vi "LIDARBrake - Rev3.vi"() -> ()   [LabVIEW 2018]
uses:
  PWFusion_TimeOfFlight_SEN-36005/LabVIEW-FRC/ToF_TypeDef/PwF ToF RangingMode.ctl
  <vilib>/Platform/TimedLoop/XDataNode/timing_clust.ctl
  <vilib>/Platform/TimedLoop/XDataNode/nitl_modes.ctl
  <vilib>/Platform/TimedLoop/XDataNode/wakeup.ctl
  <userlib>/836-Library/System/TDMS_V2/Support/TDMS_DevRef.ctl
  <userlib>/836-Library/System/TDMS_V2/Support/Logging_Settings.ctl
  <userlib>/836-Library/System/TDMS_V2/Support/Group_FIFO_Config.ctl
  <userlib>/836-Library/System/TDMS_V2/Support/Channel_FIFO_Config.ctl
  <vilib>/addons/control/pid/pid.llb/PID (DBL).vi
  <vilib>/platform/TimedLoop/XDataNode/XDataNode.xnode
  <vilib>/Platform/TimedLoop/XDataNode/XDNodeRunTimeDep.lvlib
  <vilib>/addons/control/pid/NI_PID_pid.lvlib
panel:
  out "RangingStatus":u8
  in  "LIDAR CF":dbl=1.0
  in  "x":dbl=-56.0
  in  "Reset 2":bool=TRUE
  out "Diag 2":cluster{dbl, dbl, i16}(graph)={-218.49922960069443, 18.330708661417322, 0}
  in  "Reset":bool=TRUE
  out "Diag":cluster{i32, i16, dbl, i16}(graph)={1, 0, 4.5, 0}
  in  "Read Enable":T1={"Cal Status"=TRUE, "Orientation"=TRUE, "Gyro"=FALSE, "Accelerometer"=FALSE, "Quanterion"=FALSE, "Accel Mode"=enum."Linear", "Magnetometer"=FALSE, "Register Mode"=enum."Quaternion"}
  in  "Tab Control":enum32{"Sonar", "LIDAR"}(tab)=enum."LIDAR"
  in  "Tol (sec)":dbl=0.25 format="%#_13g"
  in  "Tol (in)":dbl=1.1
  out "Arrived":bool
  out "Sonar Error":dbl=-3.3307086614173222
  in  "Rate Thresh":dbl=100.0 format="%#_13g"
  out "OOR":bool
  out "Mode":bool=TRUE
  in  "hi limit":dbl=200.0
  out "Strobe":bool
  in  "standoff":dbl=15.0 format="%.2f"
  out "Sonar Left":cluster{"Filtered":dbl, dbl}(graph)={"Filtered"=18.330708661417322, 18.330708661417322}
  out "LIDAR Late?":bool
  out "Period":i64=60
  in  "Reset Enc":bool
  out "Enc":dbl=162.49922960069443
  in  "Hyster":dbl=0.1 format="%#_13g"
  out "State":i32=1
  in  "reset IMU":bool
  in  "Test?":bool=TRUE
  in  "clamp":cluster{"output high":dbl, "output low":dbl}={"output high"=1.0, "output low"=-1.0} {"output low" format="%.2f"; "output high" format="%.2f"}
  in  "Trans":dbl=30.0
  out "close":bool=TRUE
  in  "PID Sonar":T2={"proportional gain (Kc)"=0.035, "integral time (Ti, min)"=0.0, "derivative time (Td, min)"=0.001} {"derivative time (Td, min)" format="%.5f"; "integral time (Ti, min)" format="%.3f"; "proportional gain (Kc)" format="%.3f"}
  in  "Use Enc?":bool
  out "Sonar PID":cluster{"setpoint":dbl, "Filtered":dbl, i16}(graph)={"setpoint"=15.0, "Filtered"=60.0, 0}
  out "PID error":dbl=45.0
  in  "scale enc":dbl=-0.04
  in  "db":dbl
  out "Inches 2":dbl(slide)=18.330708661417322 scale=0.0..90.0
  out "Inches":dbl(slide)=18.330708661417322 scale=0.0..90.0
  out "LIDAR (in)":dbl=18.330708661417322
  out "State 2":i32=1
  out "LIDAR Stable":bool
  in  "LIDAR Stable 2":dbl format="%#_13g"
  in  "Desired  Sample Rate ms 2":u16=50
  in  "Desired Range Mode 2":T3=enum."Medium (2m)"
  in  "RS LIDAR":bool
  in  "threshold":dbl=10.0 format="%#_13g"
  # "Real Time Data Repair"
  # "Pre-Filter"
  # "Post-Filter"
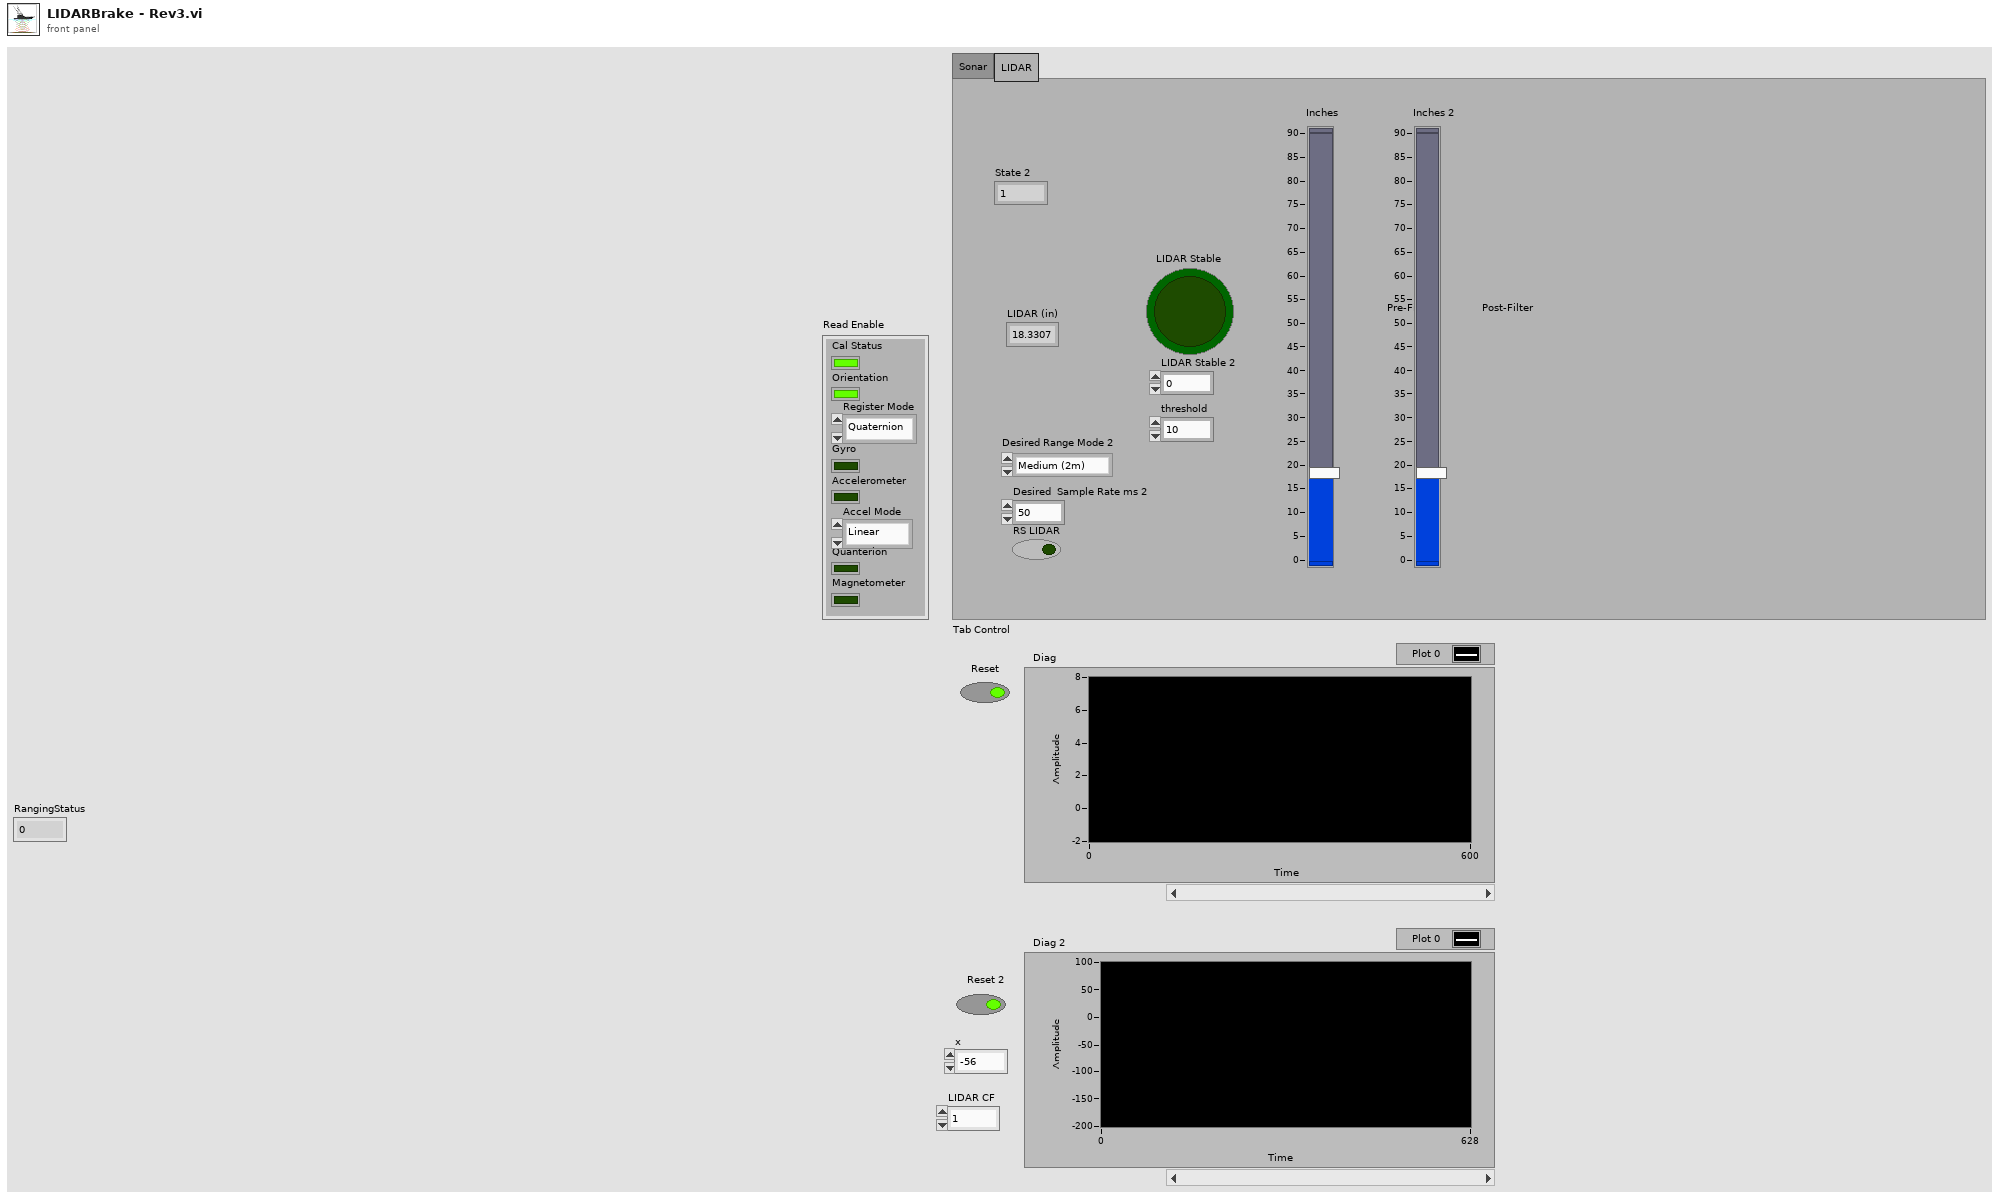
[diagram p1: front panel]
types:
  T1 = cluster{"Cal Status":bool, "Orientation":bool, "Gyro":bool, "Accelerometer":bool, "Quanterion":bool, "Accel Mode":enum8{"Raw Data", "Linear", "Gravity"}, "Magnetometer":bool, "Register Mode":enum8{"Euler", "Quaternion"}}
  T2 = cluster{"proportional gain (Kc)":dbl, "integral time (Ti, min)":dbl, "derivative time (Td, min)":dbl}
  T3 = typedef "PwF ToF RangingMode.ctl" = enum8{"Short (1.3m)", "Medium (2m)", "Long (4m)"}
  T4 = typedef "ImuDevRef.ctl" = cluster{"I2CDevRef":T5, "Valid Cal File?":bool}
  T5 = typedef "WPI_I2CDevRef.ctl" = cluster{"DevStatus":errorcluster, "Device Address":u8, "Handle":i32, "I2C Bus":T6}
  T6 = typedef "i2c_bus.ctl" = enum16{"I2C On-Board", "I2C MXP", "Invalid"}
  T7 = typedef "XDNodeRunTimeDep.lvlib/timing_clust.ctl" = cluster{"Expected End [f-1]":u64, "Actual End [f-1]":u64, "Finished Late? [f-1]":bool, "Expected End [i-1]":u64, "Actual End [i-1]":u64, "Finished Late? [i-1]":bool, "Expected Start [i]":u64, "Actual Start [i]":u64, "Expected Start [f]":u64, "Actual Start [f]":u64, "Source Name":string, "Structure Name":string, "Period":i64, "Deadline":i64, "Offset":i64, "Start":i64, "Priority":i32, "Timeout":i32, "Mode":T8, "Wakeup Reason":T9, "Error":errorcluster, "Source Type":string, "Secondary Source Type":string, "Global End Time":u64, "Global Start Time":u64, "Frame Duration":u64, "Iteration Duration":u64, "Assigned CPU":i32, "I/O Scan Engine Mode":u32}
  T8 = typedef "XDNodeRunTimeDep.lvlib/nitl_modes.ctl" = enum32{"No Change", "Process missed periods, maintain original phase", "Discard missed periods, maintain original phase", "Process missed periods, ignore original phase", "Discard missed periods, ignore original phase"}
  T9 = typedef "XDNodeRunTimeDep.lvlib/wakeup.ctl" = enum32{"Normal", "Aborted", "Asynchronous wakeup", "Timing source error", "Timed loop error", "Timeout"}
  T10 = typedef "PwF ToF Ref.ctl" = cluster{"Device ID":u8, "Ranging Mode":T3, "RefNumName":string}
  T11 = typedef "TDMS_DevRef.ctl" = cluster{"Name":string, "File Ref":refnum<k34>, "Start Time":timestamp, "Logging Settings":T12, "Group FIFO Config":T13[], "Data To Write":refnum<data-value>, "semaphore":T15, "Ref Time Reset":refnum<k4>}
  T12 = typedef "Logging_Settings.ctl" = cluster{"Data Grab Period":dbl, "File Write Period":dbl, "Max Stored Size":dbl, "Burst Size":dbl}
  T13 = typedef "Group_FIFO_Config.ctl" = cluster{"Group":string, "Channels":T14[], "Channel Names":string[]}
  T14 = typedef "Channel_FIFO_Config.ctl" = cluster{"Channel":string, "FIFO":refnum<k33>}
  T15 = typedef "Semaphore RefNum" = refnum<k1>
  T16 = cluster{"Yaw":dbl, "Roll":dbl, "Pitch":dbl, "Yaw Wind":dbl, "Roll Wind":dbl, "Pitch Wind":dbl}
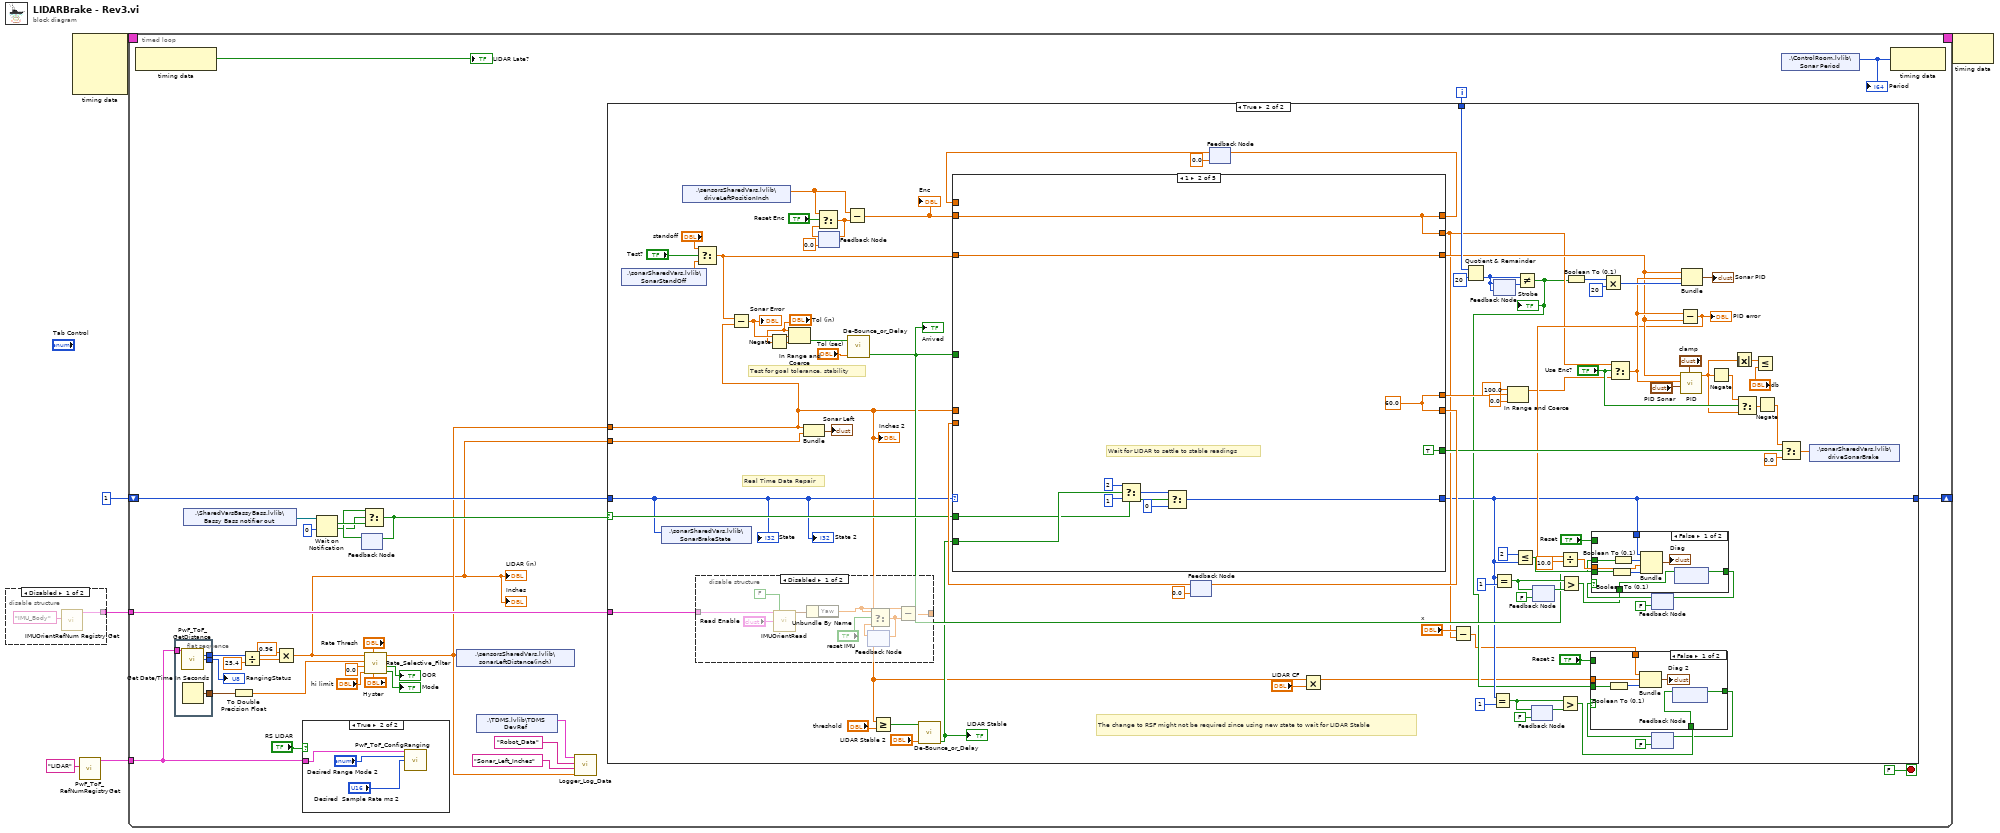
[diagram p0: block diagram]
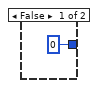
[diagram p4: hidden frame]
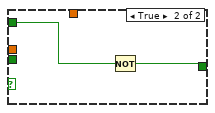
[diagram p5: hidden frame]
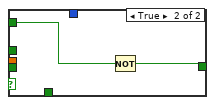
[diagram p6: hidden frame]
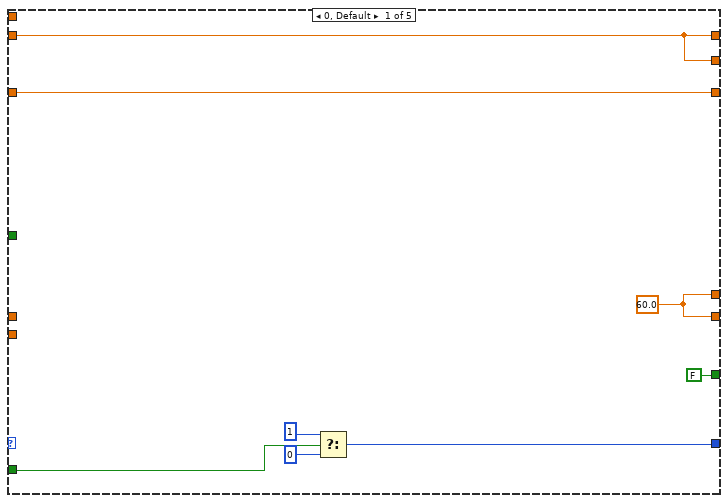
[diagram p8: hidden frame]
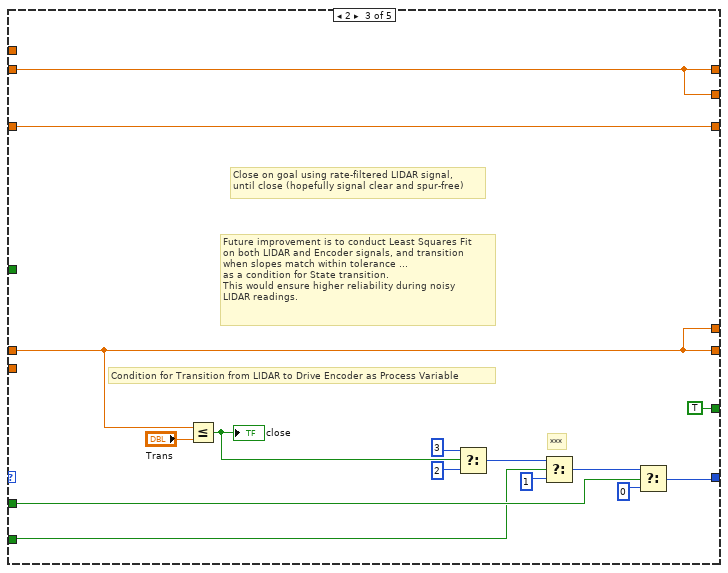
[diagram p9: hidden frame]
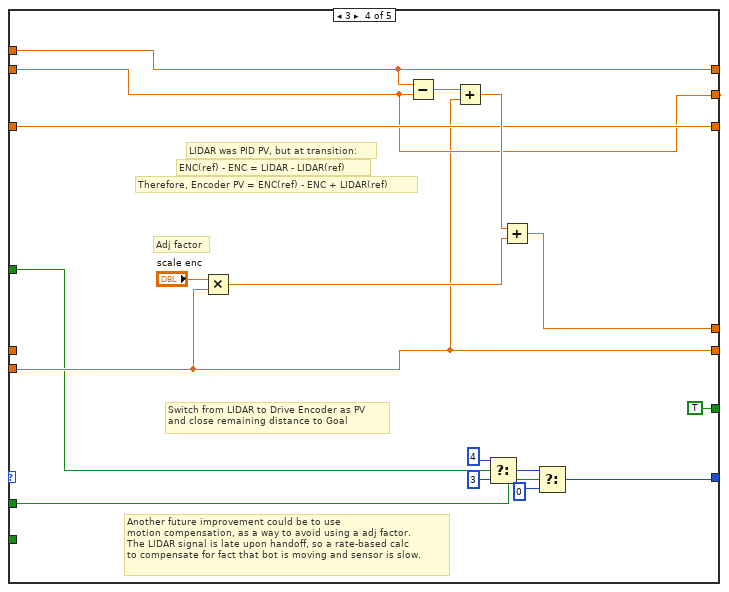
[diagram p10: hidden frame]
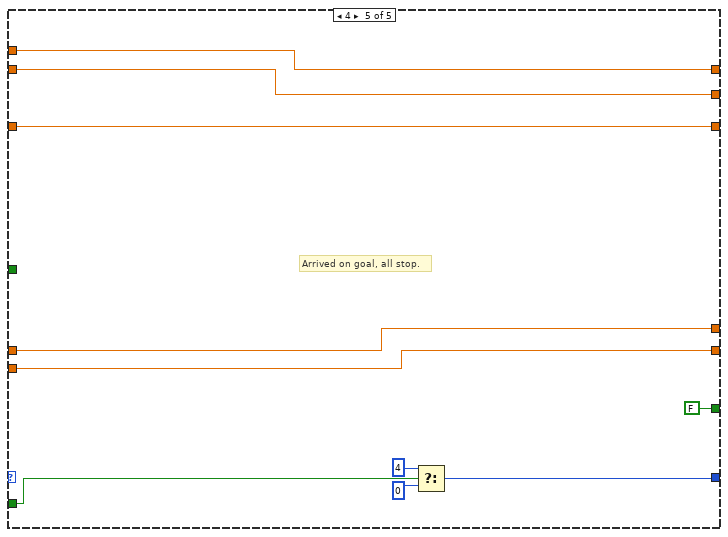
[diagram p11: hidden frame]
diagram:
  n1 = disable-structure shown="Disabled" {
    disable-tunnel: [w7 _] -> w3
    frame Disabled {
      n2 = call <userlib>:"IMUOrientRefNum Registry Get.vi"("refnum name"="IMU_Body") -> ("IMUDevRef out"=w7:T4)  [unwired: 9 in, 1 out]
    }
    frame Enabled {
    }
  }
  n3 = node-c288() -> (w6:T7)  [unwired: 4 in]
  n4 = call "PwF_ToF_RefNumRegistryGet.vi"("refnum name"="LIDAR") -> ("PwF ToF Ref"=w1:T10)  [unwired: 9 in, 1 out]
  n5 = timed-loop {
    timing: w6 -> [_]
    timing-out: [_] -> w5
    shift-right: [w35] -> _
    shift-left: 1 -> [w36]
    tunnel: w3 -> [w37]
    tunnel: w1 -> [w22]
    i -> [w39]
    stop <- FALSE stop-if-true
    n6 = node-c288() -> (→"LIDAR Late?":bool)  [unwired: 1 in]
    n7 = flat-sequence {
      tunnel: [w45] -> w27
      tunnel: [w44] -> w26
      tunnel: w22 -> [w43]
      tunnel: [w42] -> w18
      frame #0 {
        n8 = call "PwF_ToF_GetDistance.vi"("PwF ToF Ref"=w43) -> ("Dist_mm"=w44:u16, "RangingStatus"=w45:u8)  [unwired: 9 in, 4 out]
        n9 = Get Date/Time In Seconds() -> (seconds since 1Jan1904=w42:timestamp)
      }
    }
    n10 = shared-variable ".\\SharedVarsBassyBass.lvlib\\Bassy Bass notifier out"() -> (w34:refnum<notifier>)  [unwired: 1 in, 1 out]
    n11 = To Double Precision Float(number=w18) -> (double precision float=w11:dbl)
    n12 = Divide(x=w26, y=25.4) -> (x/y=w24:dbl)
    n13 = Multiply(x=0.96, y=w24) -> (x*y=w9:dbl)
    "LIDAR (in)" <- w9
    "Inches" <- w9
    n14 = case shown="True" "RS LIDAR" {
      tunnel: w22 -> [_ w46]
      frame False {
      }
      frame True {
        n15 = call "PwF_ToF_ConfigRanging.vi"("PwF ToF Ref"=w46, "Ranging Mode"="Desired Range Mode 2", "Tsamp_ms"="Desired  Sample Rate ms 2") -> ()  [unwired: 11 in, 2 out]
      }
    }
    n16 = Wait on Notification(notifier=w34, timeout in ms (-1)=0) -> (notification=w32:bool, timed out?=w30:bool)  [unwired: 2 in, 2 out]
    n17 = feedback #1() -> (w31:bool)  [unwired: 1 in]
    n18 = Select(t=w31, s=w30, f=w32) -> (s? t:f=w29:bool)
    n19 = feedback-in #1(w29) -> ()
    n20 = call <userlib>:"Rate_Selective_Filter.vi"("Hyster"="Hyster", "Rate Thresh"="Rate Thresh", "hi limit"="hi limit", "lo limit"=0.0, "Time"=w11, "Distance"=w9) -> ("Mode"=→"Mode":bool, "OOR"=→"OOR":bool, "Filtered"=w10:dbl)  [unwired: 1 in]
    n21 = shared-variable ".\\sensorsSharedVars.lvlib\\sonarLeftDistance(inch)"(w10) -> ()  [unwired: 1 in, 1 out]
    n22 = shared-variable ".\\TDMS.lvlib\\TDMS DevRef"() -> (w19:T11)  [unwired: 1 in, 1 out]
    n23 = call <userlib>:"Logger_Log_Data.vi"("Data"=w10, "Channel"="Sonar_Left_Inches", "Group"="Robot_Data", "TDMS DevRef"=w19) -> ()  [unwired: 7 in, 1 out]
    n24 = case shown="True" w29 {
      selector: w29 -> [_ w85]
      tunnel: w39 -> [_ w134]
      tunnel: w37 -> [_ w125]
      tunnel: w36 -> [_ w57]
      tunnel: [0 ("t") w62] -> w35
      tunnel: w10 -> [_ w52]
      tunnel: w9 -> [_ w51]
      frame False {
      }
      frame True {
        # "The change to RSF might not be required since using new state to wait for LIDAR Stable"
        # "Real Time Data Repair"
        # "Test for goal tolerance, stability"
        n25 = shared-variable ".\\sonarSharedVars.lvlib\\SonarStandOff"() -> (w123:dbl)  [unwired: 1 in, 1 out]
        n26 = shared-variable ".\\sonarSharedVars.lvlib\\SonarBrakeState"(w57) -> ()  [unwired: 1 in, 1 out]
        n27 = shared-variable ".\\sensorsSharedVars.lvlib\\driveLeftPositionInch"() -> (w78:dbl)  [unwired: 1 in, 1 out]
        n28 = disable-structure shown="Disabled" {
          disable-tunnel: w125 -> [w159 _]
          disable-tunnel: [w158 _] -> _
          frame Disabled {
            n29 = call <userlib>:"IMUOrientRead.vi"("IMU Dev Ref"=w159, "Orient Reset (Wind)"=FALSE, "Read Enable"="Read Enable") -> ("Orient Y/R/P"=w164:T16)  [unwired: 5 in, 7 out]
            n30 = Unbundle By Name(w164) -> ("Yaw"=w160:dbl)
            n31 = feedback #2() -> (w163:dbl)  [unwired: 1 in]
            n32 = Select(t=w160, s="reset IMU", f=w163) -> (s? t:f=w162:dbl)
            n33 = feedback-in #2(w162) -> ()
            n34 = Subtract(x=w160, y=w162) -> (x-y=w158:dbl)
          }
          frame Enabled {
          }
        }
        n35 = Select(t="standoff", s="Test?", f=w123) -> (s? t:f=w79:dbl)
        n36 = Subtract(x=w79, y=w52) -> (x-y=w133:dbl)
        "Sonar Error" <- w133
        n37 = Negate(x="Tol (in)") -> (-x=w132:dbl)
        n38 = In Range and Coerce(upper limit="Tol (in)", x=w133, lower limit=w132) -> (In Range?=w80:bool)  [unwired: 1 out]
        n39 = Bundle("Filtered"=w52, w51) -> (→"Sonar Left":cluster{"Filtered":dbl, dbl})  [unwired: 1 in]
        n40 = feedback #3(0.0) -> (w128:dbl)
        n41 = Select(t=w78, s="Reset Enc", f=w128) -> (s? t:f=w126:dbl)
        n42 = feedback-in #3(w126) -> ()
        n43 = Subtract(x=w78, y=w126) -> (x-y=w127:dbl)
        "Enc" <- w127
        n44 = call <userlib>:"De-Bounce_or_Delay.vi"("Eval Period (sec)"="Tol (sec)", "Signal Input"=w80) -> ("Stable"=w81:bool)  [unwired: 9 in]
        "Arrived" <- w81
        n45 = Greater Or Equal?(x=w52, y="threshold") -> (x >= y?=w55:bool)
        n46 = call <userlib>:"De-Bounce_or_Delay.vi"("Eval Period (sec)"="LIDAR Stable 2", "Signal Input"=w55) -> ("Stable"=w54:bool)  [unwired: 9 in]
        "LIDAR Stable" <- w54
        n47 = feedback #4(0.0 ("Filtered")) -> (w107:dbl)
        n48 = feedback #5(0.0) -> (w110:dbl)
        n49 = case shown="1" w57 {
          tunnel: [w173 w184 w200 w216 w219] -> w62
          tunnel: w85 -> [w171 w179 w199 w215 w218]
          tunnel: w79 -> [w170 w177 w194 w206 w224]
          tunnel: w127 -> [w168 w176 w192 w205 w225]
          tunnel: w52 -> [_ _ w191 _ w223]
          tunnel: w81 -> [_ _ _ w202 _]
          tunnel: [w168 w176 w192 w207 w226] -> w112
          tunnel: [w170 w177 w194 w206 w224] -> w89
          tunnel: [w167 w175 w191 w203 w222] -> w109
          tunnel: [w167 w175 w191 w204 w223] -> w76
          tunnel: [w168 w176 w192 w205 w225] -> w63
          tunnel: w110 -> [_ _ _ w207 w226]
          tunnel: w107 -> [_ _ _ w203 w222]
          tunnel: [FALSE TRUE TRUE TRUE FALSE] -> w103
          tunnel: w54 -> [_ w180 w187 _ _]
          frame 0, Default {
            w167 = 60.0
            n50 = Select(t=1, s=w171, f=0) -> (s? t:f=w173:i32)
          }
          frame 1 {
            w175 = 60.0
            # "Wait for LIDAR to settle to stable readings"
            n51 = Select(t=2, s=w180, f=1) -> (s? t:f=w181:i32)
            n52 = Select(t=w181, s=w179, f=0) -> (s? t:f=w184:i32)
          }
          frame 2 {
            # "***"
            # "Close on goal using rate-filtered LIDAR signal,\nuntil close (hopefully signal clear and spur-free)"
            # "Future improvement is to conduct Least Squares Fit\non both LIDAR and Encoder signals, and transition\nwhen slopes match within tolerance ...\nas a condition for State transition.\nThis would ensure higher reliability during noisy\nLIDAR readings."
            # "Condition for Transition from LIDAR to Drive Encoder as Process Variable"
            n53 = Less Or Equal?(x=w191, y="Trans") -> (x <= y?=w186:bool)
            "close" <- w186
            n54 = Select(t=3, s=w186, f=2) -> (s? t:f=w188:i32)
            n55 = Select(t=w188, s=w187, f=1) -> (s? t:f=w196:i32)
            n56 = Select(t=w196, s=w199, f=0) -> (s? t:f=w200:i32)
          }
          frame 3 {
            # "Adj factor"
            # "Another future improvement could be to use \nmotion compensation, as a way to avoid using a adj factor.\nThe LIDAR signal is late upon handoff, so a rate-based calc\nto compensate for fact that bot is moving and sensor is slow."
            # "Switch from LIDAR to Drive Encoder as PV\nand close remaining distance to Goal"
            # "LIDAR was PID PV, but at transition:"
            # "Therefore, Encoder PV = ENC(ref) - ENC + LIDAR(ref)"
            # "ENC(ref) - ENC = LIDAR - LIDAR(ref)"
            n57 = Multiply(x="scale enc", y=w203) -> (x*y=w211:dbl)
            n58 = Subtract(x=w207, y=w205) -> (x-y=w214:dbl)
            n59 = Add(x=w214, y=w203) -> (x+y=w212:dbl)
            n60 = Select(t=4, s=w202, f=3) -> (s? t:f=w208:i32)
            n61 = Add(x=w212, y=w211) -> (x+y=w204:dbl)
            n62 = Select(t=w208, s=w215, f=0) -> (s? t:f=w216:i32)
          }
          frame 4 {
            # "Arrived on goal, all stop."
            n63 = Select(t=4, s=w218, f=0) -> (s? t:f=w219:i32)
          }
        }
        n64 = feedback-in #4(w109) -> ()
        n65 = feedback-in #5(w112) -> ()
        n66 = Multiply(x=w52, y="LIDAR CF") -> (x*y=w59:dbl)
        n67 = Subtract(x="x", y=w63) -> (x-y=w60:dbl)
        n68 = Quotient & Remainder(x=w134, y=20) -> (floor(x/y)=w137:i32)  [unwired: 1 out]
        n69 = Equal?(x=w62, y=1) -> (x = y?=w72:bool)
        n70 = Equal?(x=w62, y=1) -> (x = y?=w95:bool)
        n71 = feedback #6(w137) -> (w136:i32)
        n72 = feedback-in #6(w137) -> ()
        n73 = In Range and Coerce(upper limit=100.0, x=w76, lower limit=0.0) -> (coerced(x)=w77:dbl)  [unwired: 1 out]
        n74 = Less Or Equal?(x=2, y=w62) -> (x <= y?=w91:bool)
        n75 = Not Equal?(x=w137, y=w136) -> (x != y?=w61:bool)
        "Strobe" <- w61
        n76 = feedback #7(FALSE ("Shock")) -> (w70:bool)
        n77 = feedback-in #7(w72) -> ()
        n78 = feedback #8(FALSE ("Shock")) -> (w97:bool)
        n79 = feedback-in #8(w95) -> ()
        n80 = Greater?(x=w72, y=w70) -> (0:w71:bool)
        n81 = Greater?(x=w95, y=w97) -> (0:w96:bool)
        n82 = Boolean To (0,1)(Boolean=w61) -> (0, 1=w119:i16)
        n83 = Multiply(x=w119, y=i16 20) -> (x*y=w115:i16)
        n84 = Select(t=w63, s="Use Enc?", f=w77) -> (s? t:f=w90:dbl)
        n85 = feedback #9(FALSE) -> (w99:bool)
        n86 = feedback #10(FALSE) -> (w68:bool)
        n87 = case shown="False" w68 {
          tunnel: "Reset 2" -> [_ w146]
          tunnel: [w143 w145] -> w67
          tunnel: w71 -> [w142 _]
          tunnel: w60 -> [w141 _]
          tunnel: w59 -> [w140 _]
          tunnel: w61 -> [w139 _]
          frame False {
            n88 = Boolean To (0,1)(Boolean=w139) -> (0, 1=w138:i16)
            n89 = Bundle(w141, w140, w138) -> (→"Diag 2":cluster{dbl, dbl, i16})  [unwired: 1 in]
            n90 = feedback #11() -> (w143:bool)  [unwired: 1 in]
            n91 = feedback-in #11(w142) -> ()
          }
          frame True {
            n92 = Not(x=w146) -> (.not. x?=w145:bool)
          }
        }
        n93 = feedback-in #10(w67) -> ()
        n94 = Subtract(x=w90, y=w89) -> (x-y=w88:dbl)
        "PID error" <- w88
        n95 = Divide(x=w88, y=10.0) -> (x/y=w93:dbl)
        n96 = case shown="False" w99 {
          tunnel: w62 -> [w154 _]
          tunnel: w81 -> [w152 _]
          tunnel: w93 -> [w151 _]
          tunnel: "Reset" -> [_ w157]
          tunnel: [w150 w156] -> w87
          tunnel: w96 -> [w149 _]
          tunnel: w91 -> [w147 _]
          frame False {
            n97 = Boolean To (0,1)(Boolean=w147) -> (0, 1=w148:i16)
            n98 = Boolean To (0,1)(Boolean=w152) -> (0, 1=w153:i16)
            n99 = Bundle("t"=w154, w153, w151, w148) -> (→"Diag":cluster{"t":i32, i16, dbl, i16})  [unwired: 1 in]
            n100 = feedback #12() -> (w150:bool)  [unwired: 1 in]
            n101 = feedback-in #12(w149) -> ()
          }
          frame True {
            n102 = Not(x=w157) -> (.not. x?=w156:bool)
          }
        }
        n103 = feedback-in #9(w87) -> ()
        n104 = call-poly <vilib>:"PID.vi"("output range"="clamp", "PID gains"="PID Sonar", "process variable"=w90, "setpoint"=w89) -> ("output"=w84:dbl)  [unwired: 6 in, 1 out]
        n105 = Bundle("Double"=w89, "upper limit"=w90, w115) -> (→"Sonar PID":cluster{"Double":dbl, "upper limit":dbl, i16})  [unwired: 1 in]
        n106 = Negate(x=w84) -> (-x=w114:dbl)
        n107 = Absolute Value(x=w84) -> (abs(x)=w83:dbl)
        n108 = Select(t=w114, s="Use Enc?", f=w84) -> (s? t:f=w86:dbl)
        n109 = Less Or Equal?(x=w83, y="db") -> ()  [unwired: 1 out]
        n110 = Negate(x=w86) -> (-x=w106:dbl)
        n111 = Select(t=w106, s=w103, f=0.0) -> (s? t:f=w105:dbl)
        n112 = shared-variable ".\\sonarSharedVars.lvlib\\driveSonarBrake"(w105) -> ()  [unwired: 1 in, 1 out]
        "State" <- w57
        "Inches 2" <- w52
        "State 2" <- w57
      }
    }
    n113 = shared-variable ".\\ControlRoom.lvlib\\Sonar Period"() -> (w38:i64)  [unwired: 1 in, 1 out]
    "Period" <- w38
    n114 = node-c288(w38) -> ()  [unwired: 1 out]
    "RangingStatus" <- w27
  }
  n115 = node-c288(w5) -> ()  [unwired: 1 out]
